vi "Get Session Running Status.vi"(8 "error in (no error)":errorcluster, 11 "Engine Simulation IP in":refnum<class "Engine Simulation IP.lvclass">) -> (0 "error out":errorcluster, 2 "running":bool, 3 "Engine Simulation IP out":refnum<class "Engine Simulation IP.lvclass">)   [LabVIEW 2013, in "Engine Simulation IP.lvclass"]
uses:
  Engine Simulation IP.lvclass
  Engine Simulation IP.lvclass/Engine Simulation IP.ctl
  Engine Simulation Session.lvclass/Engine Simulation Session.ctl
  Engine Simulation Session.lvclass
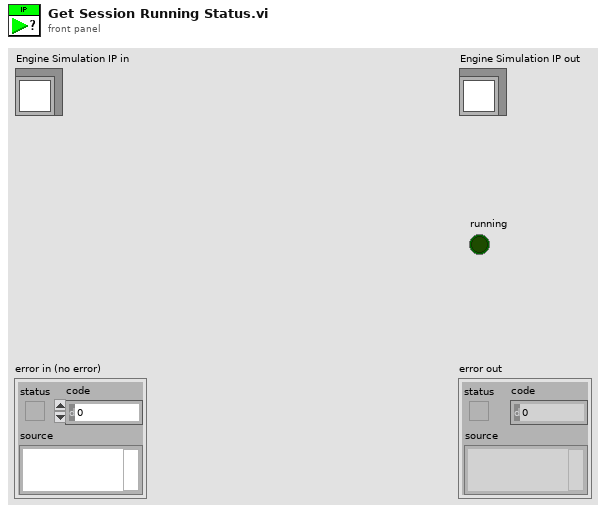
[diagram p1: front panel]
types:
  T1 = typedef "Engine Simulation IP.lvclass/IP class private data.ctl" = cluster{"Name":string, "EST version enum":T2, "session":refnum<class "Engine Simulation Session.lvclass">}
  T2 = typedef "Engine Simulation Session.lvclass/Bitfile Major Version.ctl" = enum16{"1.0", "1.1", "1.2", "1.3"}
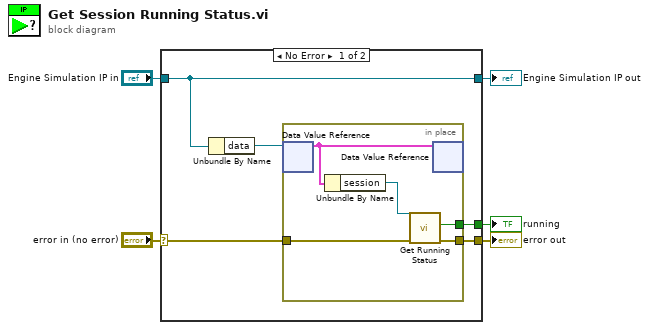
[diagram p0: block diagram]
diagram:
  n1 = case shown="No Error" "error in (no error)" {
    selector: "error in (no error)" -> [w10 w17]
    tunnel: [w9 w17] -> w4
    tunnel: [w8 w16] -> w2
    tunnel: "Engine Simulation IP in" -> [w8 w16]
    tunnel: [w6 _] -> w1
    frame No Error {
      n2 = Unbundle By Name(w8) -> ("data"=w7:refnum<data-value>)
      n3 = in-place {
        in-place-border: w10 -> [w15]
        in-place-border: [w14] -> w9
        in-place-border: [w11] -> w6
        n4 = in-place-dvr #1(w7) -> (w13:T1)  [unwired: 1 out]
        n5 = Unbundle By Name(w13) -> ("session"=w12:refnum<class "Engine Simulation Session.lvclass">)
        n6 = call "Get Running Status.vi"("error in (no error)"=w15, "Engine Simulation Session in"=w12) -> ("error out"=w14:errorcluster, "running"=w11:bool)  [unwired: 7 in, 1 out]
        n7 = in-place-dvr #1(w13) -> ()  [unwired: 2 out]
      }
    }
    frame Error {
    }
  }
  "error out" <- w4
  "Engine Simulation IP out" <- w2
  "running" <- w1
